vi "Tribe Logger.vi"(8 "error in (no error)":errorcluster) -> (0 "error out":errorcluster)   [LabVIEW 2023]
uses:
  <vilib>/Utility/config.llb/Config Data RefNum.ctl
  acca670c-cdbf-466a-a659-b8260685f3aa.vi
  <userlib>/_MGI/Application Control/MGI Gray if/MGI Gray if False.vi
  <vilib>/Utility/config.llb/Read Key (String).vi
  <vilib>/Utility/config.llb/NI_LVConfig.lvlib
panel:
  in  "Log Chat?":bool
  in  "Map":string(combo)
  in  "Start/Stop":bool
  in  "Post Interval":i32=15 min=1 max=1000
  in  "Exit":bool
  # "minutes"
  # "Remember to disable\nAuto-Hide if you turn\non chat logging"
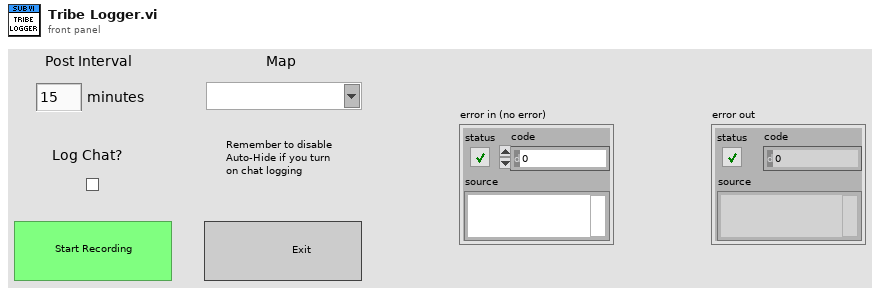
[diagram p1: front panel]
types:
  T1 = enum8{"Enabled", "Disabled", "Disabled and Grayed Out"}
  T2 = enum32{"Invalid", "Standard", "Closed", "Hidden", "Minimized", "Maximized"}
  T3 = enum32{"invalid app kind", "Development System", "Run Time System", "Student Edition", "Embedded LabVIEW", "Evaluation", "Custom"}
  T4 = typedef "NI_LVConfig.lvlib/Config Data RefNum.ctl" = refnum<k1>
  T5 = cluster{"Core":cluster{"Current VI Reference":refnum<vi>, "Close Panel on Exit?":bool}, "last":timestamp, "image":path, "Config":T4}
  T6 = cluster{"Current VI Reference":refnum<vi>, "Close Panel on Exit?":bool}
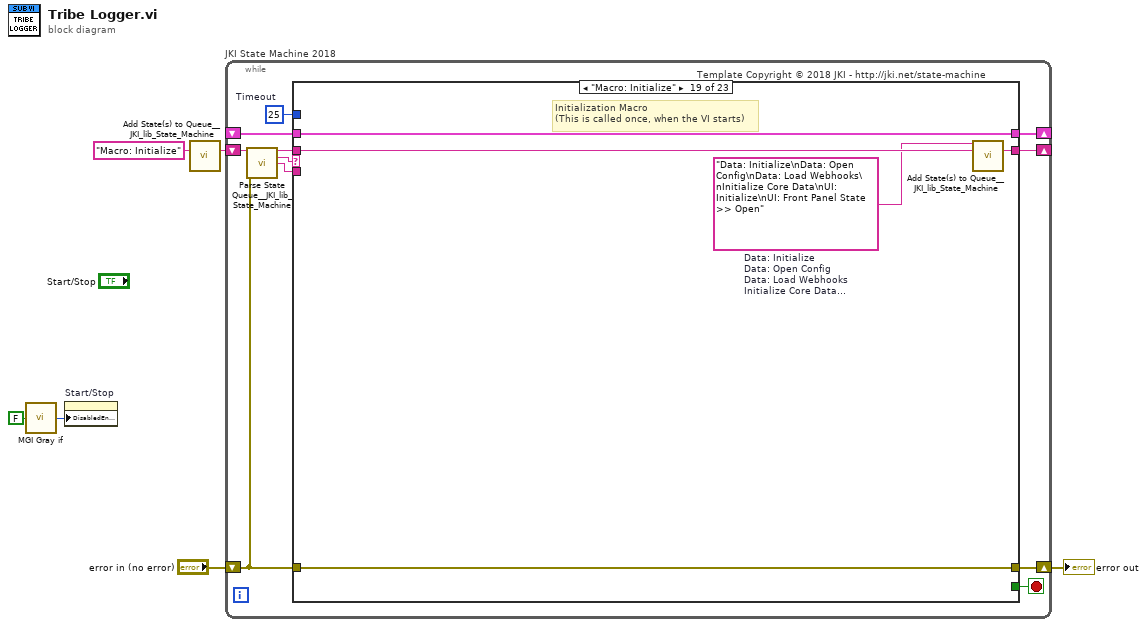
[diagram p0: block diagram]
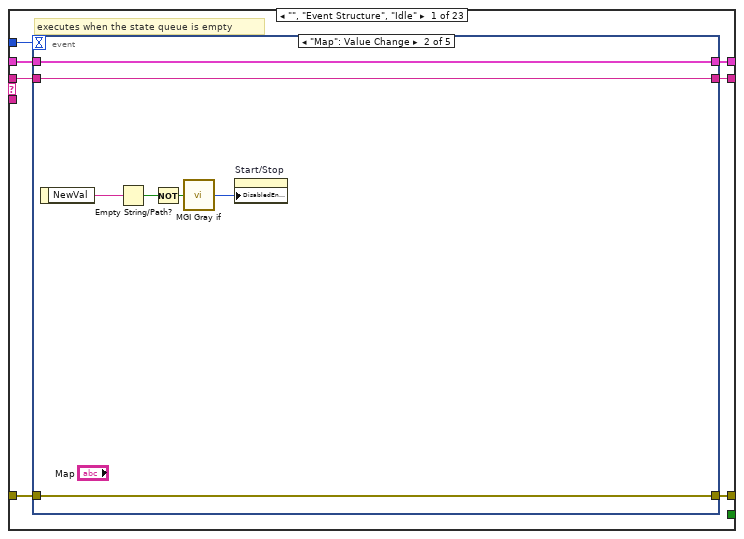
[diagram p2: hidden frame]
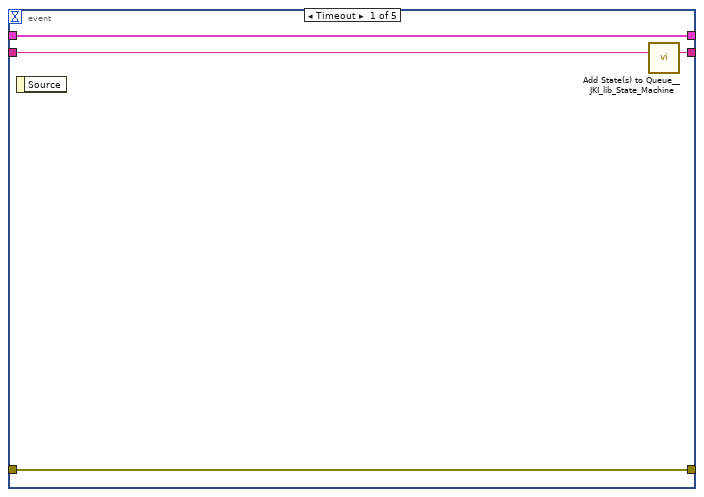
[diagram p3: hidden frame]
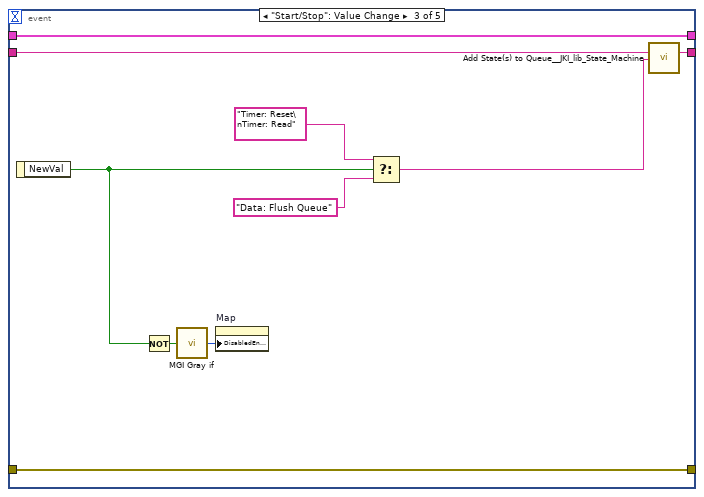
[diagram p4: hidden frame]
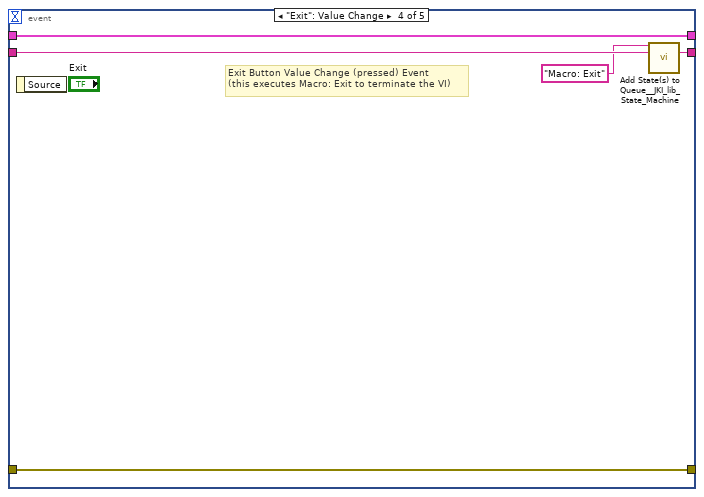
[diagram p5: hidden frame]
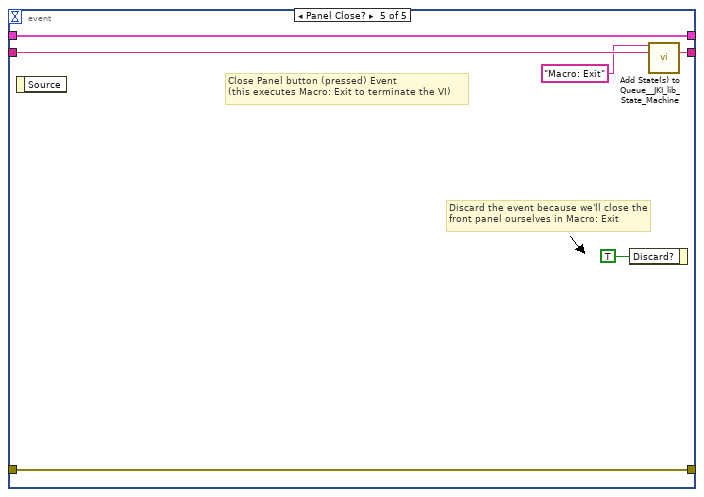
[diagram p6: hidden frame]
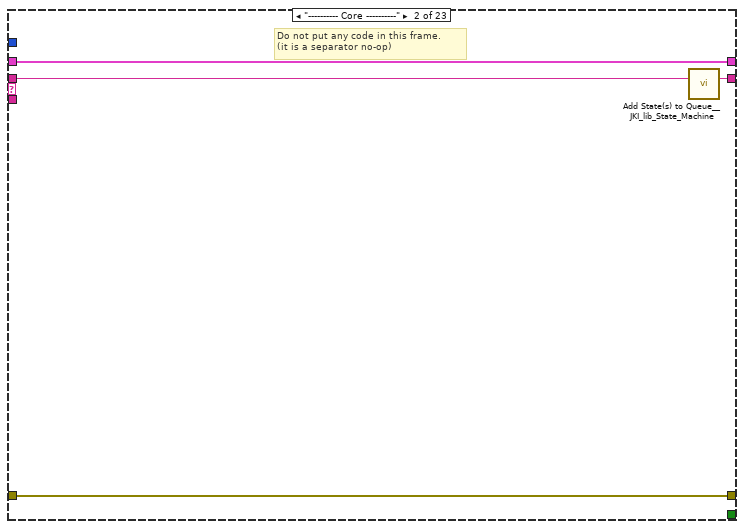
[diagram p7: hidden frame]
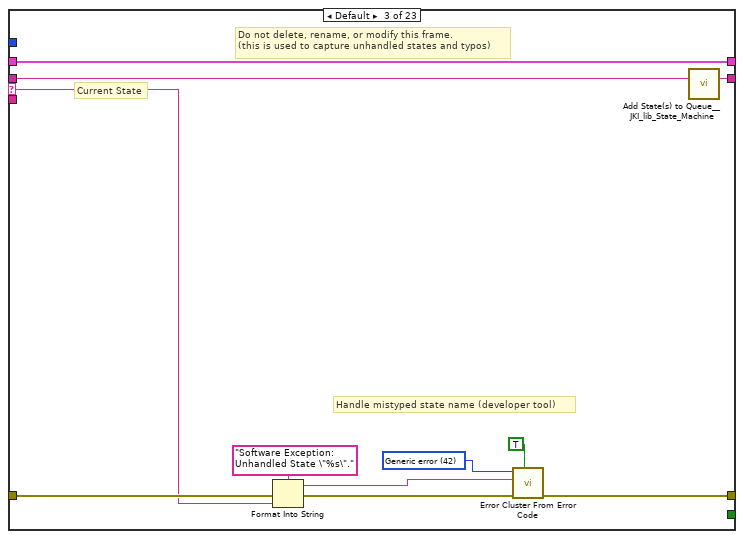
[diagram p8: hidden frame]
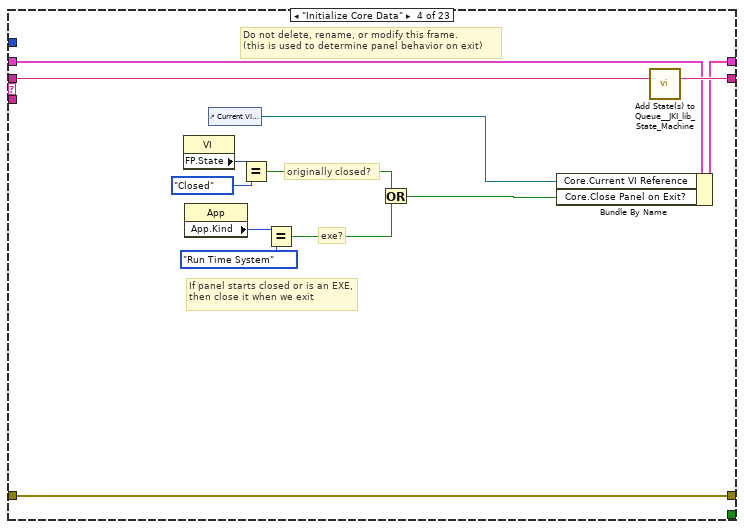
[diagram p9: hidden frame]
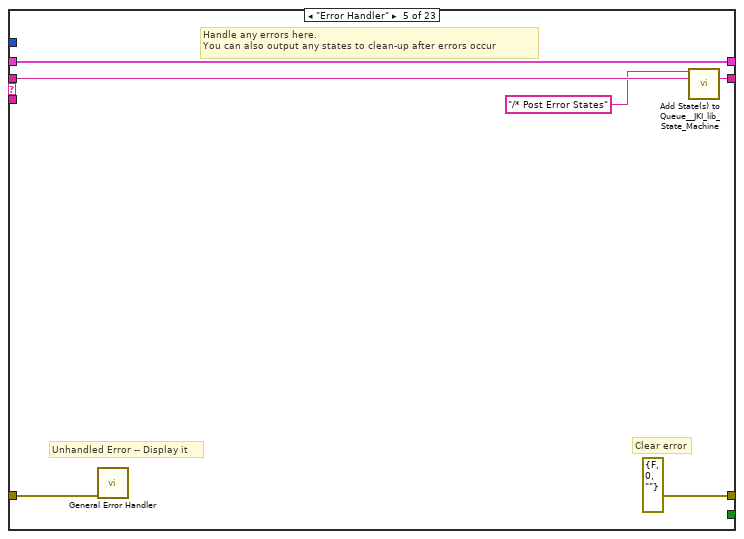
[diagram p10: hidden frame]
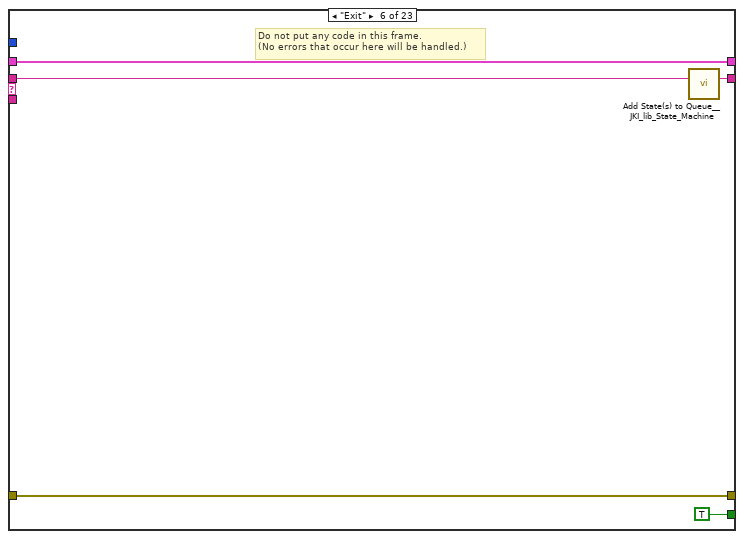
[diagram p11: hidden frame]
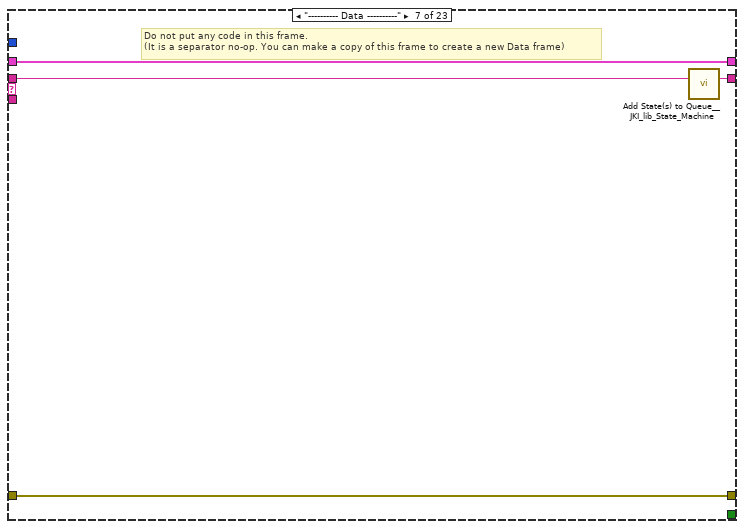
[diagram p12: hidden frame]
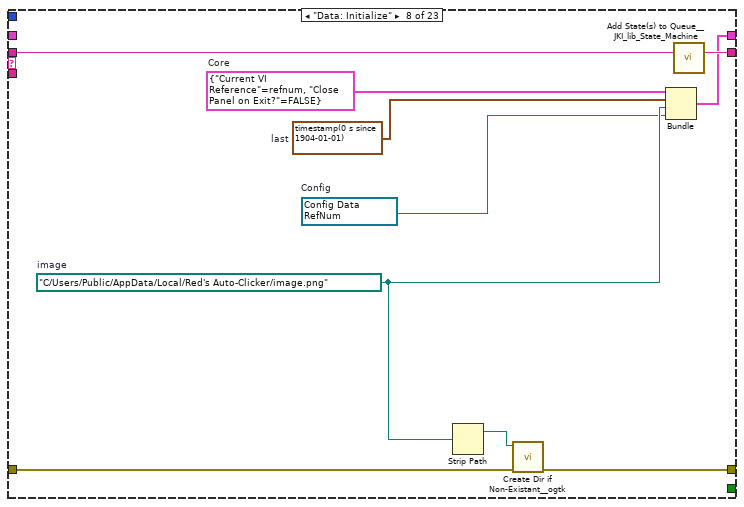
[diagram p13: hidden frame]
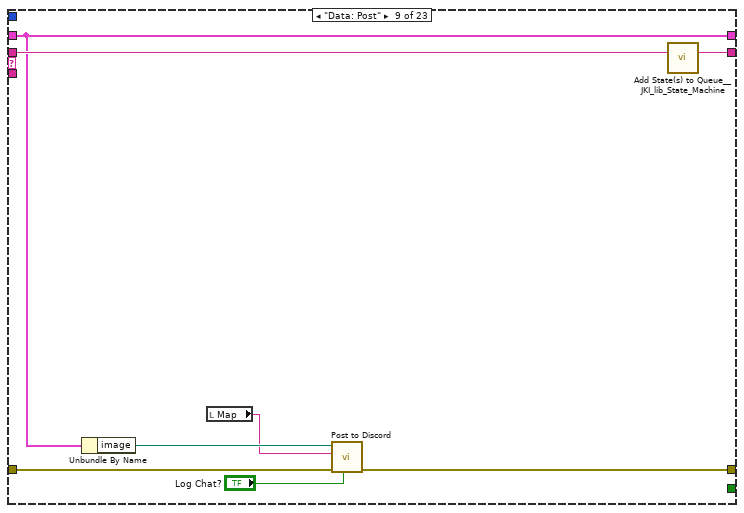
[diagram p14: hidden frame]
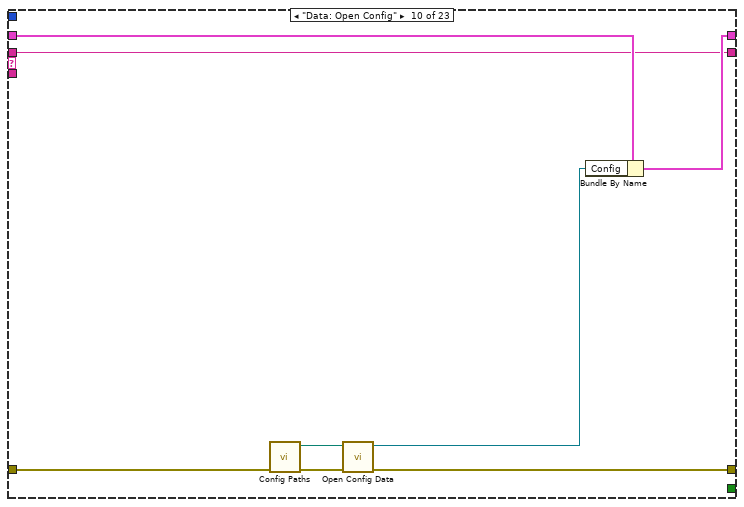
[diagram p15: hidden frame]
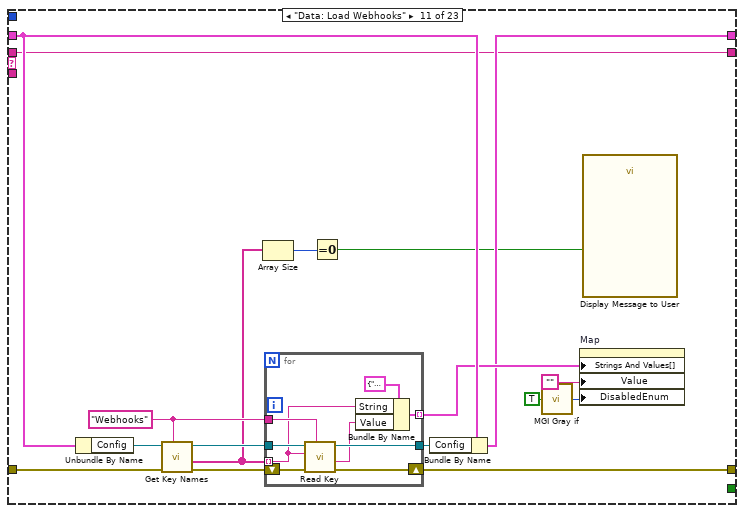
[diagram p16: hidden frame]
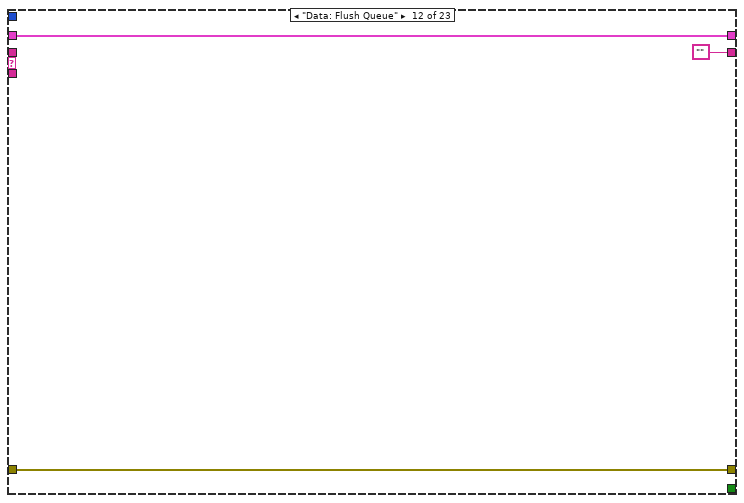
[diagram p17: hidden frame]
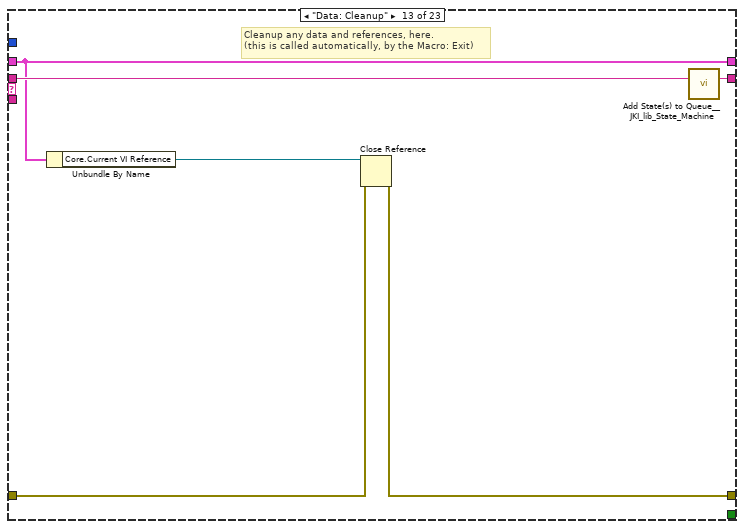
[diagram p18: hidden frame]
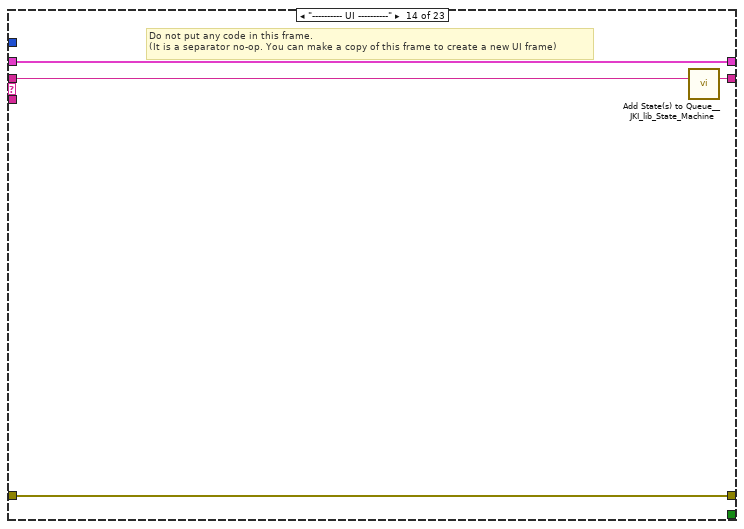
[diagram p19: hidden frame]
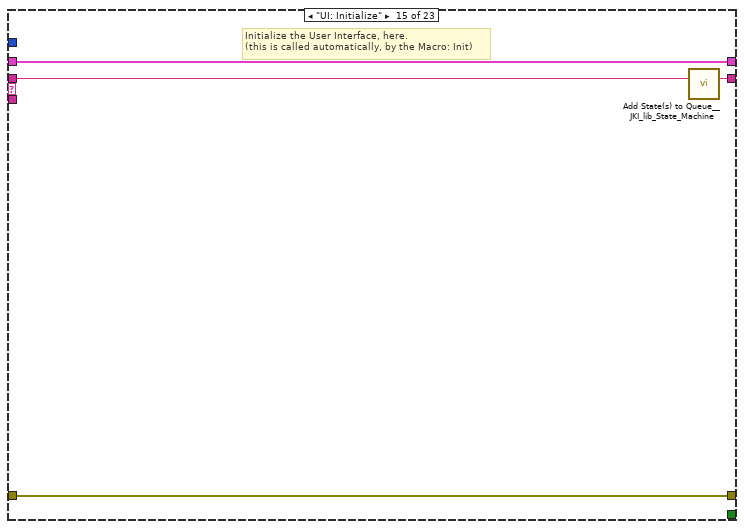
[diagram p20: hidden frame]
diagram:
  n1 = call-poly <userlib>:"MGI Gray if.vi"("Boolean"=FALSE) -> ("Disabled"=w3:T1)
  n2 = property on="Start/Stop" class="Bool (strict)"("DisabledEnum"=w3) -> ()  [unwired: 2 in, 2 out]
  n3 = call <vilib>:"Add State(s) to Queue__JKI_lib_State_Machine.vi"("State(s) in (\"\")"="Macro: Initialize") -> ("States Out"=w6:string)  [unwired: 14 in]
  n4 = while "JKI State Machine 2018" {
    shift-right: [w10] -> _
    shift-left: _ -> [w9]
    shift-right: [w13] -> w2
    shift-left: "error in (no error)" -> [w7]
    shift-right: [w12] -> _
    shift-left: w6 -> [w14]
    stop <- w11 stop-if-true
    w8 = 25  # Timeout
    # "Template Copyright © 2018 JKI - http://jki.net/state-machine"
    n5 = call <vilib>:"Parse State Queue__JKI_lib_State_Machine.vi"("State Queue"=w14, "Error In (no error)"=w7) -> ("Remaining States"=w16:string, "Current State"=w17:string, "Arguments"=w15:string)  [unwired: 11 in]
    n6 = case shown="\"Macro: Initialize\"" w17 {
      selector: w17 -> [_ _ w61 _ _ _ _ _ _ _ _ _ _ _ _ _ _ _ _ _ _ _ _]
      tunnel: w16 -> [w24 w60 w65 w84 w90 w95 w99 w109 w117 w120 w130 _ w160 w164 w168 w174 w185 w254 w259 w269 w273 w289 w295]
      tunnel: w15 -> [_ _ _ _ _ _ _ _ _ _ _ _ _ _ _ w169 w179 _ _ _ _ _ _]
      tunnel: w9 -> [w22 w57 w63 w77 w87 w93 w96 _ w111 w122 w136 w154 w155 w161 w166 w172 w181 w251 w256 w266 w270 w284 w292]
      tunnel: [w21 w58 w67 w81 errorcluster {"status"=FALSE, "code"=0, "source"=""} ("error out") w92 w97 w102 w114 w118 w129 w152 w156 w162 w165 w170 w182 w252 w257 w267 w271 w277 w293] -> w13
      tunnel: w7 -> [w20 w58 w66 w81 w86 w92 w97 w103 w115 w123 w138 w152 w157 w162 w165 w171 w183 w252 w257 w267 w271 w287 w293]
      tunnel: [w23 w59 w64 w83 w89 w94 w98 w108 w116 w120 w130 "" w159 w163 w167 w173 w184 w253 w258 w268 w272 w288 w294] -> w12
      tunnel: [_ _ _ _ _ TRUE _ _ _ _ _ _ _ _ _ _ _ _ _ _ _ _ _] -> w11
      tunnel: [w19 w57 w63 w82 w87 w93 w96 w107 w111 w121 w131 w154 w155 w161 w166 w172 w181 w251 w256 w266 w270 w284 w291] -> w10
      tunnel: w8 -> [w18 _ _ _ _ _ _ _ _ _ _ _ _ _ _ _ _ _ _ _ _ _ _]
      frame "", "Event Structure", "Idle" {
        # "executes when the state queue is empty"
        n7 = event shown="[1] \"Map\": Value Change" {
          selector: _ -> [_ _ _ _ _]
          dyn-events: _ -> [_ _ _ _ _]
          timeout: w18 -> [_ _ _ _ _]
          tunnel: w24 -> [w28 w29 w45 w50 w56]
          tunnel: [w27 w29 w44 w49 w55] -> w23
          tunnel: w22 -> [w25 w30 w42 w47 w53]
          tunnel: [w26 w35 w43 w48 w54] -> w21
          tunnel: w20 -> [w26 w35 w43 w48 w54]
          tunnel: [w25 w30 w42 w47 w53] -> w19
          event Timeout {
            n8 = event-data() -> ()  [unwired: 1 in, 1 out]
            n9 = call <vilib>:"Add State(s) to Queue__JKI_lib_State_Machine.vi"("State(s) in (\"\")"=w28) -> ("States Out"=w27:string)  [unwired: 14 in]
          }
          event "Map": Value Change {
            n10 = event-data() -> ("NewVal"=w34:string)  [unwired: 1 in]
            n11 = Empty String/Path?(string/path=w34) -> (empty?=w33:bool)
            n12 = Not(x=w33) -> (.not. x?=w32:bool)
            n13 = call-poly <userlib>:"MGI Gray if.vi"("Boolean"=w32) -> ("Disabled"=w31:T1)
            n14 = property on="Start/Stop" class="Bool (strict)"("DisabledEnum"=w31) -> ()  [unwired: 2 in, 2 out]
          }
          event "Start/Stop": Value Change {
            n15 = event-data() -> ("NewVal"=w38:bool)  [unwired: 1 in]
            n16 = Not(x=w38) -> (.not. x?=w37:bool)
            n17 = call-poly <userlib>:"MGI Gray if.vi"("Boolean"=w37) -> ("Disabled"=w36:T1)
            n18 = property on="Map" class="CmbBox"("DisabledEnum"=w36) -> ()  [unwired: 2 in, 2 out]
            n19 = Select(t="Timer: Reset\nTimer: Read", s=w38, f="Data: Flush Queue") -> (s? t:f=w39:string)
            n20 = call <vilib>:"Add State(s) to Queue__JKI_lib_State_Machine.vi"("State(s) in (\"\")"=w45, "State(s) at Back (\"\")"=w39) -> ("States Out"=w44:string)  [unwired: 13 in]
          }
          event "Exit": Value Change {
            # "Exit Button Value Change (pressed) Event\n(this executes Macro: Exit to terminate the VI)"
            n21 = event-data() -> ()  [unwired: 1 in, 1 out]
            n22 = call <vilib>:"Add State(s) to Queue__JKI_lib_State_Machine.vi"("State(s) in Front (\"\")"="Macro: Exit", "State(s) in (\"\")"=w50) -> ("States Out"=w49:string)  [unwired: 13 in]
          }
          event Panel Close? {
            # "Discard the event because we'll close the front panel ourselves in Macro: Exit"
            # "Close Panel button (pressed) Event\n(this executes Macro: Exit to terminate the VI)"
            n23 = event-data() -> ()  [unwired: 1 in, 1 out]
            n24 = event-data("Discard?"=TRUE) -> ()  [unwired: 1 in, 1 out]
            n25 = call <vilib>:"Add State(s) to Queue__JKI_lib_State_Machine.vi"("State(s) in Front (\"\")"="Macro: Exit", "State(s) in (\"\")"=w56) -> ("States Out"=w55:string)  [unwired: 13 in]
          }
        }
      }
      frame "---------- Core ----------" {
        # "Do not put any code in this frame.\n(it is a separator no-op)"
        n26 = call <vilib>:"Add State(s) to Queue__JKI_lib_State_Machine.vi"("State(s) in (\"\")"=w60) -> ("States Out"=w59:string)  [unwired: 14 in]
      }
      frame Default {
        w70 = 42 items=["No error", "Argument error", "Memory is full", "Out of zone", "End of file", "File already open", "Generic file I/O error", "File not found", "File permission error", "Disk is full", "Duplicate path", "Too many files open", "System feature not enabled", "Resource file not found", "Cannot add resource", "Resource not found", "Image not found", "Image memory error", "Pen does not exist", "Config type invalid", "Config token not found", "Config parse error", "Config memory error", "Bad external code format", "Bad external code offset", "External code not present", "Null window", "Destroy window error", "Null menu", "Print aborted", "Bad print record", "Print driver error", "Windows error during printing", "Memory error during printing", "Print dialog error", "Generic print error", "Invalid device refnum", "Device not found", "Device parameter error", "Device unit error", "Cannot open device", "Device call aborted", "Generic error", "Cancelled by user", "Object ID too low", "Object ID too high", "Object not in heap", "Unknown heap", "Unknown object (invalid DefProc)", "Unknown object (DefProc not in table)", "Message out of range", "Invalid (null) method", "Unknown message", "Manager call not supported", "Bad address", "Network operation in progress", "Network operation timed out", "Connection is busy", "Network attribute not supported", "Network error", "Address in use", "System out of memory", "Connection aborted", "Connection refused", "Not connected", "Already connected", "Connection closed", "Initialization error (interapplication manager)", "Bad occurrence", "Wait on unbound occurrence handler", "Occurrence queue overflow", "Datalog type conflict", "Unused", "Unrecognized type (interapplication manager)", "Memory corrupt", "Failed to make temporary DLL", "Old CIN version", "Drag socket not found", "Failed to load drop-object", "Failed to register OLE object", "Failed to release OLE object", "Format specifier type mismatch", "Unknown format specifier", "Too few format specifiers", "Too many format specifiers", "Scan failed", "Newer CIN version", "Error converting to variant", "Runtime menu error", "Password tampered", "Variant attribute not found", "Incompatible variant data type", "Event data is not available", "Event Store is not present", "Occurrence is not found", "Event Queue is not created", "Event info is not available", "Refnum passed is NULL", "Error retrieving Class GUID", "Error retrieving CoClass GUID", "Error retrieving TypeLib GUID.", "Bad built application magic bytes.", "Specific driver is different from the specific driver associated with the Logical Name.", "There is no session opened to the class driver.", "Max Error", "MAX - Error with config objects", "MAX - Error loading configuration", "MAX - Group not supported"]
        # "Current State"
        # "Do not delete, rename, or modify this frame.\n(this is used to capture unhandled states and typos)"
        # "Handle mistyped state name (developer tool)"
        n27 = Format Into String(format string="Software Exception: Unhandled State \"%s\"." ("message"), error in=w66, w61) -> (resulting string=w69:string, error out=w68:errorcluster)  [unwired: 1 in]
        n28 = call <vilib>:"Error Cluster From Error Code.vi"("show call chain? (False)"=TRUE, "error in (no error)"=w68, "error message (\"\")"=w69, "error code (0)"=w70) -> ("error out"=w67:errorcluster)  [unwired: 5 in]
        n29 = call <vilib>:"Add State(s) to Queue__JKI_lib_State_Machine.vi"("State(s) in (\"\")"=w65) -> ("States Out"=w64:string)  [unwired: 14 in]
      }
      frame "Initialize Core Data" {
        # "Do not delete, rename, or modify this frame.\n(this is used to determine panel behavior on exit)"
        # "originally closed?"
        # "exe?"
        # "If panel starts closed or is an EXE, then close it when we exit"
        n30 = property class="VI"() -> ("FP.State"=w74:T2)  [unwired: 2 in, 2 out]
        n31 = property class="App"() -> ("App.Kind"=w80:T3)  [unwired: 2 in, 2 out]
        n32 = control-ref of="Current VI Reference"() -> (w75:refnum<vi>)
        n33 = Equal?(x=w74, y=T2."Closed" ("Front Panel Window:State")) -> (x = y?=w72:bool)
        n34 = Equal?(x=w80, y=T3."Run Time System" ("Application:Kind")) -> (x = y?=w78:bool)
        n35 = Or(x=w72, y=w78) -> (x .or. y?=w76:bool)
        n36 = Bundle By Name(cluster=w77, "Core.Current VI Reference"=w75, "Core.Close Panel on Exit?"=w76) -> (w82:T5)
        n37 = call <vilib>:"Add State(s) to Queue__JKI_lib_State_Machine.vi"("State(s) in (\"\")"=w84) -> ("States Out"=w83:string)  [unwired: 14 in]
      }
      frame "Error Handler" {
        # "Unhandled Error -- Display it"
        # "Handle any errors here.\nYou can also output any states to clean-up after errors occur"
        # "Clear error"
        n38 = call <vilib>:"General Error Handler.vi"("error in (no error)"=w86) -> ()  [unwired: 10 in, 5 out]
        n39 = call <vilib>:"Add State(s) to Queue__JKI_lib_State_Machine.vi"("State(s) in Front (\"\")"="/* Post Error States", "State(s) in (\"\")"=w90) -> ("States Out"=w89:string)  [unwired: 13 in]
      }
      frame "Exit" {
        # "Do not put any code in this frame.\n(No errors that occur here will be handled.)"
        n40 = call <vilib>:"Add State(s) to Queue__JKI_lib_State_Machine.vi"("State(s) in (\"\")"=w95) -> ("States Out"=w94:string)  [unwired: 14 in]
      }
      frame "---------- Data ----------" {
        # "Do not put any code in this frame.\n(It is a separator no-op. You can make a copy of this frame to create a new Data frame)"
        n41 = call <vilib>:"Add State(s) to Queue__JKI_lib_State_Machine.vi"("State(s) in (\"\")"=w99) -> ("States Out"=w98:string)  [unwired: 14 in]
      }
      frame "Data: Initialize" {
        w100 = T4 refnum items=["config data"]  # Config
        w101 = path "C:/Users/Public/AppData/Local/Red's Auto-Clicker/image.png"  # image
        w105 = timestamp(0 s since 1904-01-01)  # last
        w106 = T6 {"Current VI Reference"=refnum, "Close Panel on Exit?"=FALSE}  # Core
        n42 = Strip Path(path=w101) -> (stripped path=w104:path)  [unwired: 1 out]
        n43 = call <userlib>:"Create Dir if Non-Existant__ogtk.vi"("error in (no error)"=w103, "Directory Path"=w104) -> ("error out"=w102:errorcluster)  [unwired: 7 in, 2 out]
        n44 = Bundle("Core"=w106, "last"=w105, "image"=w101, "Config"=w100) -> (w107:T5)  [unwired: 1 in]
        n45 = call <vilib>:"Add State(s) to Queue__JKI_lib_State_Machine.vi"("State(s) in (\"\")"=w109) -> ("States Out"=w108:string)  [unwired: 14 in]
      }
      frame "Data: Post" {
        n46 = Unbundle By Name(w111) -> ("image"=w113:path)
        n47 = local read "Map"() -> (w112:string)
        n48 = call "Post to Discord.vi"("Log Chat?"="Log Chat?", "error in (no error)"=w115, "Mapppp"=w112, "Image Path"=w113) -> ("error out"=w114:errorcluster)  [unwired: 7 in]
        n49 = call <vilib>:"Add State(s) to Queue__JKI_lib_State_Machine.vi"("State(s) in (\"\")"=w117) -> ("States Out"=w116:string)  [unwired: 14 in]
      }
      frame "Data: Open Config" {
        n50 = call "Config Paths.vi"("error in (no error)"=w123) -> ("error out"=w125:errorcluster, "Global Config"=w124:path)  [unwired: 7 in, 2 out]
        n51 = call <vilib>:"Open Config Data.vi"("error in (no error)"=w125, "configuration file path"=w124) -> ("error out"=w118:errorcluster, "refnum"=w119:T4)  [unwired: 7 in, 1 out]
        n52 = Bundle By Name(cluster=w122, "Config"=w119) -> (w121:T5)
      }
      frame "Data: Load Webhooks" {
        w139 = "Webhooks" ("section")
        n53 = Unbundle By Name(w136) -> ("Config"=w142:T4)
        n54 = call <vilib>:"Get Key Names.vi"("section"=w139, "error in (no error)"=w138, "refnum"=w142) -> ("error out"=w140:errorcluster, "key names"=w128:string[], "refnum out"=w141:T4)  [unwired: 5 in, 1 out]
        n55 = Array Size(array=w128) -> (size(s)=w127:i32)
        n56 = for {
          tunnel: w141 -> [w151]
          tunnel: w128 -> [w145] mode=indexing
          tunnel: w139 -> [w149]
          shift-right: [w148] -> w129
          shift-left: w140 -> [w150]
          tunnel: [w147] -> w137
          tunnel: [w143] -> w132 mode=indexing
          n57 = call-poly <vilib>:"Read Key.vi"("section"=w149, "error in (no error)"=w150, "key"=w145, "refnum"=w151) -> ("error out"=w148:errorcluster, "value"=w144:string, "refnum out"=w147:T4)  [unwired: 4 in, 1 out]
          n58 = Bundle By Name(cluster=cluster{"String":string, "Value":string} {"String"="", "Value"=""} ("Cluster"), "String"=w145, "Value"=w144) -> (w143:cluster{"String":string, "Value":string})
        }
        n59 = Equal To 0?(x=w127) -> (x = 0?=w126:bool)
        n60 = Bundle By Name(cluster=w136, "Config"=w137) -> (w131:T5)
        n61 = call-poly <userlib>:"MGI Gray if.vi"("Boolean"=TRUE) -> ("Disabled"=w135:T1)
        n62 = property on="Map" class="CmbBox"("Strings And Values[]"=w132, "Value"="", "DisabledEnum"=w135) -> ()  [unwired: 2 in, 2 out]
        n63 = call "Display Message to User"("Enable"=w126) -> ()  [unwired: 9 in, 2 out]
      }
      frame "Data: Flush Queue" {
      }
      frame "Data: Cleanup" {
        # "Cleanup any data and references, here.\n(this is called automatically, by the Macro: Exit)"
        n64 = Unbundle By Name(w155) -> ("Core.Current VI Reference"=w158:refnum<vi>)
        n65 = Close Reference(reference=w158, error in (no error)=w157) -> (error out=w156:errorcluster)
        n66 = call <vilib>:"Add State(s) to Queue__JKI_lib_State_Machine.vi"("State(s) in (\"\")"=w160) -> ("States Out"=w159:string)  [unwired: 14 in]
      }
      frame "---------- UI ----------" {
        # "Do not put any code in this frame.\n(It is a separator no-op. You can make a copy of this frame to create a new UI frame)"
        n67 = call <vilib>:"Add State(s) to Queue__JKI_lib_State_Machine.vi"("State(s) in (\"\")"=w164) -> ("States Out"=w163:string)  [unwired: 14 in]
      }
      frame "UI: Initialize" {
        # "Initialize the User Interface, here.\n(this is called automatically, by the Macro: Init)"
        n68 = call <vilib>:"Add State(s) to Queue__JKI_lib_State_Machine.vi"("State(s) in (\"\")"=w168) -> ("States Out"=w167:string)  [unwired: 14 in]
      }
      frame "UI: Cursor Set" {
        # "Argument"
        # "Set and Unset Cursor Busy.\n(Usage: \"UI: Cursor Set >> Busy|Idle\")"
        n69 = case shown="\"Idle\", Default" w169 {
          tunnel: w171 -> [w176 w178]
          tunnel: [w175 w177] -> w170
          frame "Idle", Default {
            n70 = call <vilib>:"Unset Busy.vi"("error in (no error)"=w176) -> ("error out"=w175:errorcluster)  [unwired: 10 in]
          }
          frame "Busy" {
            n71 = call <vilib>:"Set Busy.vi"("error in (no error)"=w178) -> ("error out"=w177:errorcluster)  [unwired: 9 in, 1 out]
          }
        }
        n72 = call <vilib>:"Add State(s) to Queue__JKI_lib_State_Machine.vi"("State(s) in (\"\")"=w174) -> ("States Out"=w173:string)  [unwired: 14 in]
      }
      frame "UI: Front Panel State" {
        # "Argument"
        # "Set Front Panel Open or Closed\n(Usage: \"UI: Front Panel State >> Open|Close\")"
        n73 = Unbundle By Name(w181) -> ("Core.Current VI Reference"=w180:refnum<vi>)
        n74 = case shown="\"Minimize\", \"Minimized\"" w179 {
          tunnel: w183 -> [w191 w206 w217 w230 w243]
          tunnel: [w193 w207 w219 w232 w245] -> w182
          tunnel: w180 -> [w192 w204 w218 w231 w244]
          frame "Open", "Standard", Default {
            w186 = T2."Standard" ("State")
            n75 = property class="VI"(reference=w192, error in=w191) -> (reference out=w189:refnum<vi>, error out=w190:errorcluster, "FP.State"=w188:T2)
            n76 = Not Equal?(x=w188, y=w186) -> (x != y?=w187:bool)
            n77 = case shown="True" w187 {
              tunnel: [w197 w199] -> w193
              tunnel: w190 -> [w196 w199]
              tunnel: w189 -> [w195 _]
              tunnel: w186 -> [w194 _]
              frame True {
                n78 = invoke class="VI" method="FP.Open"(reference=w195, error in=w196, "Activate"=TRUE, "State"=w194) -> (error out=w197:errorcluster)  [unwired: 1 in, 4 out]
              }
              frame False {
              }
            }
          }
          frame "Close", "Closed" {
            n79 = property class="VI"(reference=w204, error in=w206) -> (reference out=w203:refnum<vi>, error out=w205:errorcluster, "FP.State"=w201:T2)
            n80 = Not Equal?(x=w201, y=T2."Closed" ("Front Panel Window:State")) -> (x != y?=w200:bool)
            n81 = case shown="True" w200 {
              tunnel: [w208 w211] -> w207
              tunnel: w205 -> [w208 w210]
              tunnel: w203 -> [_ w209]
              frame False {
              }
              frame True {
                n82 = invoke class="VI" method="FP.Close"(reference=w209, error in=w210) -> (error out=w211:errorcluster)  [unwired: 1 in, 2 out]
              }
            }
          }
          frame "Hidden", "Hide" {
            w212 = T2."Hidden" ("State")
            n83 = property class="VI"(reference=w218, error in=w217) -> (reference out=w215:refnum<vi>, error out=w216:errorcluster, "FP.State"=w214:T2)
            n84 = Not Equal?(x=w214, y=w212) -> (x != y?=w213:bool)
            n85 = case shown="True" w213 {
              tunnel: [w223 w224] -> w219
              tunnel: w216 -> [w222 w224]
              tunnel: w215 -> [w221 _]
              tunnel: w212 -> [w220 _]
              frame True {
                n86 = invoke class="VI" method="FP.Open"(reference=w221, error in=w222, "State"=w220) -> (error out=w223:errorcluster)  [unwired: 2 in, 4 out]
              }
              frame False {
              }
            }
          }
          frame "Minimize", "Minimized" {
            w225 = T2."Minimized" ("State")
            n87 = property class="VI"(reference=w231, error in=w230) -> (reference out=w228:refnum<vi>, error out=w229:errorcluster, "FP.State"=w227:T2)
            n88 = Not Equal?(x=w227, y=w225) -> (x != y?=w226:bool)
            n89 = case shown="True" w226 {
              tunnel: [w236 w237] -> w232
              tunnel: w229 -> [w235 w237]
              tunnel: w228 -> [w234 _]
              tunnel: w225 -> [w233 _]
              frame True {
                n90 = invoke class="VI" method="FP.Open"(reference=w234, error in=w235, "State"=w233) -> (error out=w236:errorcluster)  [unwired: 2 in, 4 out]
              }
              frame False {
              }
            }
          }
          frame "Maximize", "Maximized" {
            w238 = T2."Maximized" ("State")
            n91 = property class="VI"(reference=w244, error in=w243) -> (reference out=w241:refnum<vi>, error out=w242:errorcluster, "FP.State"=w240:T2)
            n92 = Not Equal?(x=w240, y=w238) -> (x != y?=w239:bool)
            n93 = case shown="True" w239 {
              tunnel: [w249 w250] -> w245
              tunnel: w242 -> [w248 w250]
              tunnel: w241 -> [w247 _]
              tunnel: w238 -> [w246 _]
              frame True {
                n94 = invoke class="VI" method="FP.Open"(reference=w247, error in=w248, "State"=w246) -> (error out=w249:errorcluster)  [unwired: 2 in, 4 out]
              }
              frame False {
              }
            }
          }
        }
        n95 = call <vilib>:"Add State(s) to Queue__JKI_lib_State_Machine.vi"("State(s) in (\"\")"=w185) -> ("States Out"=w184:string)  [unwired: 14 in]
      }
      frame "---------- Macro ----------" {
        # "Do not put any code in this frame.\n(It is a separator no-op. You can make a copy of this frame to create a new Macro frame)"
        n96 = call <vilib>:"Add State(s) to Queue__JKI_lib_State_Machine.vi"("State(s) in (\"\")"=w254) -> ("States Out"=w253:string)  [unwired: 14 in]
      }
      frame "Macro: Initialize" {
        w255 = "Data: Initialize\nData: Open Config\nData: Load Webhooks\nInitialize Core Data\nUI: Initialize\nUI: Front Panel State >> Open"  # Data: Initialize Data: Open Config Data: Load Webhooks Initialize Core Data UI: Initialize UI: Front Panel State >> Open
        # "Initialization Macro\n(This is called once, when the VI starts)"
        n97 = call <vilib>:"Add State(s) to Queue__JKI_lib_State_Machine.vi"("State(s) in Front (\"\")"=w255, "State(s) in (\"\")"=w259) -> ("States Out"=w258:string)  [unwired: 13 in]
      }
      frame "Macro: Exit" {
        # "Exit Macro\n(This is called once, when the VI exits)"
        n98 = Unbundle By Name(w266) -> ("Core.Close Panel on Exit?"=w265:bool)
        n99 = Select(t="UI: Front Panel State >> Close", s=w265, f="") -> (s? t:f=w262:string)
        n100 = call <vilib>:"Add State(s) to Queue__JKI_lib_State_Machine.vi"("State(s) in (\"\")"=w262, "State(s) at Back (\"\")"="Data: Cleanup\nExit") -> ("States Out"=w260:string)  [unwired: 13 in]
        n101 = call <vilib>:"Add State(s) to Queue__JKI_lib_State_Machine.vi"("State(s) in Front (\"\")"=w260, "State(s) in (\"\")"=w269) -> ("States Out"=w268:string)  [unwired: 13 in]
      }
      frame "---------- Timer ----------" {
        # "Template Separator\n(You can make a copy of, or modify, this frame)"
        n102 = call <vilib>:"Add State(s) to Queue__JKI_lib_State_Machine.vi"("State(s) in (\"\")"=w273) -> ("States Out"=w272:string)  [unwired: 14 in]
      }
      frame "Timer: Read" {
        n103 = Multiply(x="Post Interval", y=60.0) -> (x*y=w280:dbl)
        n104 = Unbundle By Name(w284) -> ("last"=w282:timestamp)
        n105 = Get Date/Time In Seconds() -> (seconds since 1Jan1904=w283:timestamp)
        n106 = Subtract(x=w283, y=w282) -> (x-y=w281:dbl)
        n107 = Greater Or Equal?(x=w281, y=w280) -> (x >= y?=w279:bool)
        n108 = call "Stall Data Flow.vim"("value in"=w287, "milliseconds to wait"=u32 100) -> ("value out"=w277:errorcluster)  [unwired: 1 out]
        n109 = Select(t="Timer: Reset\nData: Post\nTimer: Read", s=w279, f="Idle\nTimer: Read") -> (s? t:f=w274:string)
        n110 = call <vilib>:"Add State(s) to Queue__JKI_lib_State_Machine.vi"("State(s) in (\"\")"=w289, "State(s) at Back (\"\")"=w274) -> ("States Out"=w288:string)  [unwired: 13 in]
      }
      frame "Timer: Reset" {
        n111 = Get Date/Time In Seconds() -> (seconds since 1Jan1904=w290:timestamp)
        n112 = Bundle By Name(cluster=w292, "last"=w290) -> (w291:T5)
        n113 = call <vilib>:"Add State(s) to Queue__JKI_lib_State_Machine.vi"("State(s) in (\"\")"=w295) -> ("States Out"=w294:string)  [unwired: 14 in]
      }
    }
  }
  "error out" <- w2
